vi "DriveForwardAuto.vi"   [LabVIEW 2014]
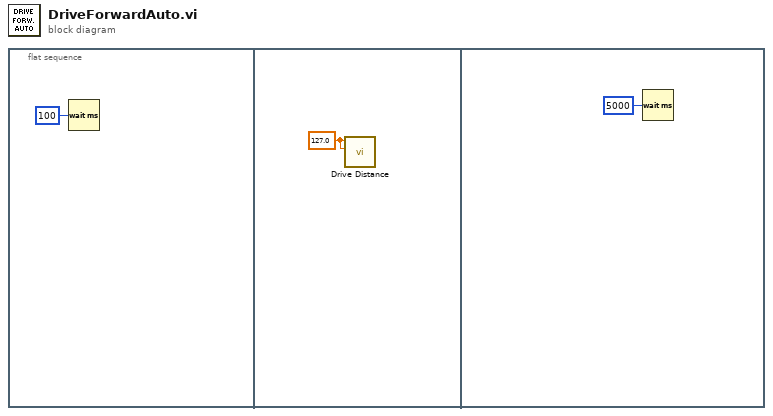
[diagram p0: block diagram]
diagram:
  n1 = flat-sequence {
    frame #0 {
      n2 = Wait (ms)(milliseconds to wait=u32 100) -> ()  [unwired: 1 out]
    }
    frame #1 {
      w2 = 127.0 ("Desired Left Inches")
      n3 = call "Drive Distance.vi"("Desired Right Inches"=w2, "Desired Left Inches"=w2) -> ()  [unwired: 10 in]
    }
    frame #2 {
      n4 = Wait (ms)(milliseconds to wait=u32 5000) -> ()  [unwired: 1 out]
    }
  }
